vi "cw_5_1.vi"() -> ()   [LabVIEW 2022 SP3]
uses:
  Dimensions_input_tdef.ctl
panel:
  in  "Dimentions":T1
  out "Area of hexahedron":dbl
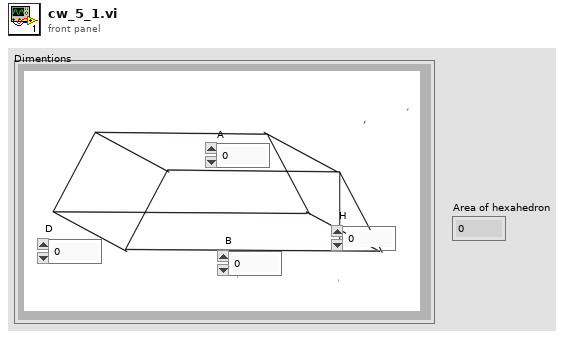
[diagram p1: front panel]
types:
  T1 = typedef "Dimensions_input_tdef.ctl" = cluster{"B":dbl, "A":dbl, "H":dbl, "D":dbl}
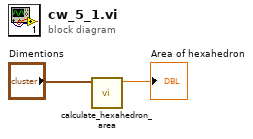
[diagram p0: block diagram]
diagram:
  n1 = call "calculate_hexahedron_area.vi"("Dimentions"="Dimentions") -> ("Area of hexahedron"=→"Area of hexahedron":dbl)  [unwired: 10 in]
